vi "Git Flow Start Hotfix.vi"(8 "error in (no error)":errorcluster, 10 "version":string, 11 "Git in":refnum<class "Git.lvclass">) -> (0 "error out":errorcluster, 2 "standard output":string, 3 "Git out":refnum<class "Git.lvclass">)   [LabVIEW 2019, in "Git.lvclass"]
uses:
  Git.lvclass
  Typedefs/Commands.git-flow--combo.ctl
  Typedefs/Branches.git-flow--combo.ctl
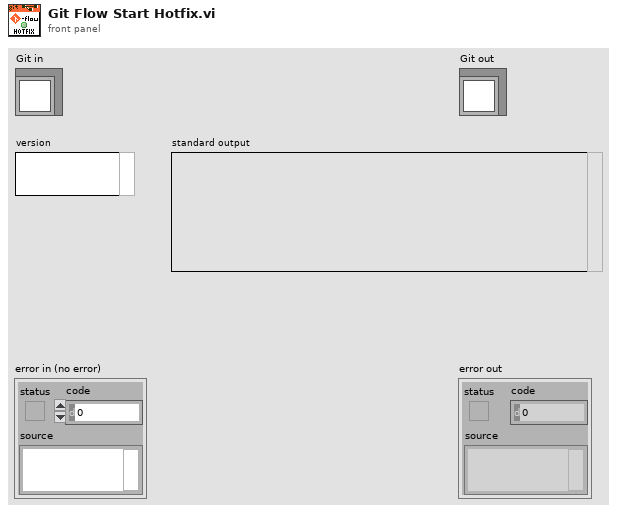
[diagram p1: front panel]
types:
  T1 = typedef "Git.lvclass/Branches.git-flow--combo.ctl" = string
  T2 = typedef "Git.lvclass/Commands.git-flow--combo.ctl" = string
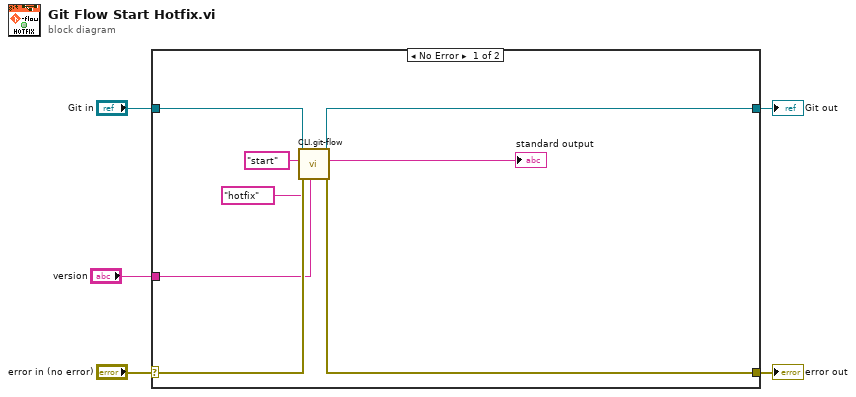
[diagram p0: block diagram]
diagram:
  n1 = case shown="No Error" "error in (no error)" {
    selector: "error in (no error)" -> [w13 w15]
    tunnel: [w12 w15] -> w4
    tunnel: [w11 w14] -> w2
    tunnel: "Git in" -> [w10 w14]
    tunnel: "version" -> [w8 _]
    frame No Error {
      n2 = call "CLI.git-flow.vi"("name"=w8, "error in (no error)"=w13, "Branch"=T1 "hotfix", "Command"=T2 "start", "Git in"=w10) -> ("error out"=w12:errorcluster, "standard output"=→"standard output":string, "Git out"=w11:refnum<class "Git.lvclass">)  [unwired: 2 in, 2 out]
    }
    frame Error {
    }
  }
  "error out" <- w4
  "Git out" <- w2
